vi "convert timespec to seconds.vi"(11 "timespec":cluster{"sec":u64, "nsec":u64}) -> (3 "seconds":dbl)   [LabVIEW 2013, in "Linux RT Utilities.lvlib"]
uses:
  Linux RT Utilities.lvlib
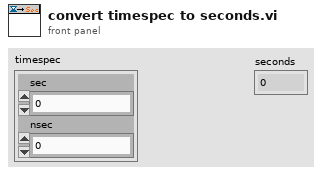
[diagram p1: front panel]
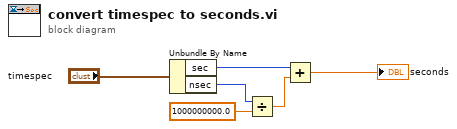
[diagram p0: block diagram]
diagram:
  n1 = Unbundle By Name("timespec") -> ("sec"=w2:u64, "nsec"=w3:u64)
  n2 = Divide(x=w3, y=1000000000.0) -> (x/y=w1:dbl)
  n3 = Add(x=w2, y=w1) -> (x+y=→"seconds":dbl)
